vi "STM Read Message.vi"   [LabVIEW 2015]
doc: "This VI reads an incoming package of data from a host. This VI parses the package and extracts the data name and type as described in the meta data.\n\nFor the package to be parsed correctly, the meta data must be consistent in both the sender and the receiver. The data is packaged based on the existing meta data on the sender. \n\nUse the \"STM Read Meta Data\" and \"STM Write Meta Data\" VIs to ensure that both client and server have the same meta data.\n\nThe data is returned as a string. It is the responsibility of the user to cast it to the appropriate type.\n\nCopyright 2015, 2016, 2017 National Instruments Corporation\n\nLicensed under the Apache License, Version 2.0 (the \"License\"); you may not use this file except in compliance with the License.\n\n You may obtain a copy of the License at\n\n http://www.apache.org/licenses/LICENSE-2.0\n\nUnless required by applicable law or agreed to in writing, software distributed under the License is distributed on an \"AS IS\" BASIS, WITHOUT WARRANTIES OR CONDITIONS OF ANY KIND, either express or implied.\n\nSee the License for the specific language governing permissions and limitations under the License."
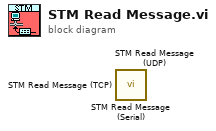
[diagram p0: block diagram]
diagram:
  n1 = call <vilib>:"STM Read Message (Serial).vi"() -> ()  [unwired: 6 in, 6 out]
  n2 = call <vilib>:"STM Read Message (UDP).vi"() -> ()  [unwired: 6 in, 6 out]
  n3 = call <vilib>:"STM Read Message (TCP).vi"() -> ()  [unwired: 6 in, 6 out]
